vi "myRIO_BRig_RT_dataExp_CueCycles.vi"() -> (2 "output_CueCycles":i32)   [LabVIEW 2014]
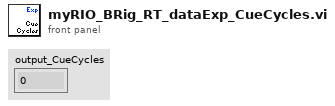
[diagram p1: front panel]
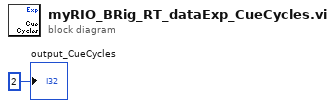
[diagram p0: block diagram]
diagram:
  "output_CueCycles" <- 2 ("output_iBlock")
